vi "testTCP.vi"() -> ()   [LabVIEW 2024]
panel:
  in  "stop":bool
  out "counter":i32
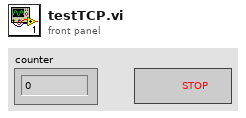
[diagram p1: front panel]
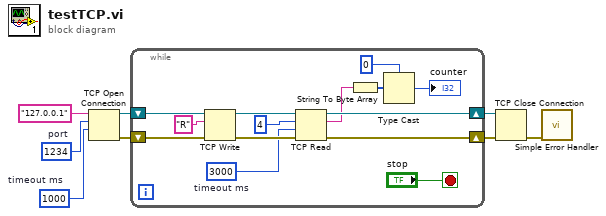
[diagram p0: block diagram]
diagram:
  w6 = 1000  # timeout ms
  w7 = u16 1234  # port
  n1 = TCP Open Connection(address="127.0.0.1", remote port or service name=w7, timeout ms (60000)=w6) -> (connection ID=w5:refnum<k5>, error out=w4:errorcluster)  [unwired: 2 in]
  n2 = while {
    shift-right: [w15] -> w2
    shift-left: w5 -> [w22]
    shift-right: [w16] -> w3
    shift-left: w4 -> [w18]
    stop <- "stop" stop-if-true
    w14 = 3000  # timeout ms
    n3 = TCP Write(connection ID=w22, data in="R", error in (no error)=w18) -> (connection ID out=w20:refnum<k5>, error out=w17:errorcluster)  [unwired: 1 in, 1 out]
    n4 = TCP Read(connection ID=w20, bytes to read=4, error in (no error)=w17, 9:w14) -> (connection ID out=w15:refnum<k5>, data out=w9:string, error out=w16:errorcluster)  [unwired: 1 in]
    n5 = String To Byte Array(string=w9) -> (unsigned byte array=w10:u8[])
    n6 = Type Cast(type=0, x=w10) -> (*(type *) &x=→"counter":i32)
  }
  n7 = TCP Close Connection(connection ID=w2, error in (no error)=w3) -> (error out=w1:errorcluster)  [unwired: 1 in, 1 out]
  n8 = call <vilib>:"Simple Error Handler.vi"("error in (no error)"=w1) -> ()  [unwired: 4 in, 5 out]
